vi "Set_PS1_15V_in_Series.vi"(3 "error in":errorcluster) -> (10 "error out":errorcluster)   [LabVIEW 2015]
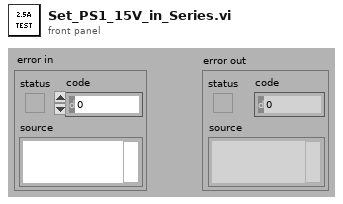
[diagram p1: front panel]
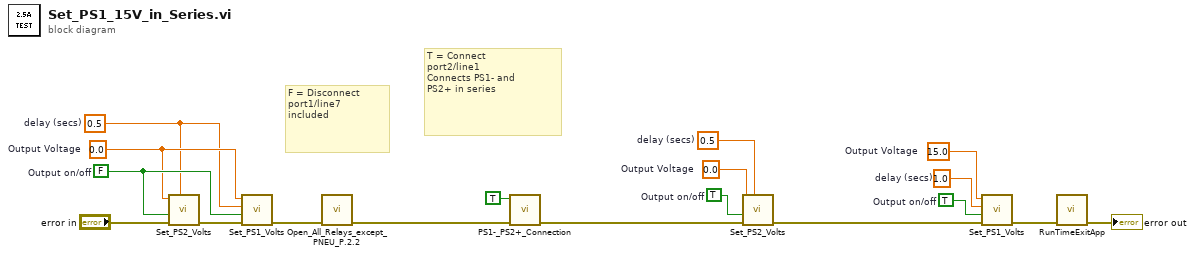
[diagram p0: block diagram]
diagram:
  w3 = TRUE  # Output on/off
  w4 = 0.5  # delay (secs)
  w5 = 0.0  # Output Voltage
  w12 = TRUE  # Output on/off
  w11 = 1.0  # delay (secs)
  w10 = 15.0  # Output Voltage
  w14 = 0.0  # Output Voltage
  w13 = 0.5  # delay (secs)
  w15 = FALSE  # Output on/off
  # "T = Connect\nport2/line1\nConnects PS1- and\nPS2+ in series"
  # "F = Disconnect\nport1/line7\nincluded"
  n1 = call "Set_PS2_Volts.vi"("delay (secs)"=w13, "error in"="error in", "Output on/off"=w15, "Output Voltage"=w14) -> ("error out"=w16:errorcluster)  [unwired: 5 in, 2 out]
  n2 = call "Set_PS1_Volts.vi"("error in"=w16, "Output on/off"=w15, "delay (secs)"=w13, "Output Voltage"=w14) -> ("error out"=w7:errorcluster)  [unwired: 5 in, 2 out]
  n3 = call "Open_All_Relays_except_PNEU_P.2.2.vi"("error in"=w7) -> ("error out"=w6:errorcluster)  [unwired: 9 in]
  n4 = call "PS1-_PS2+_Connection.vi"("On/Off"=TRUE, "error in"=w6) -> ("error out"=w2:errorcluster)  [unwired: 8 in]
  n5 = call "Set_PS2_Volts.vi"("delay (secs)"=w4, "error in"=w2, "Output on/off"=w3, "Output Voltage"=w5) -> ("error out"=w1:errorcluster)  [unwired: 5 in, 2 out]
  n6 = call "Set_PS1_Volts.vi"("error in"=w1, "Output on/off"=w12, "delay (secs)"=w11, "Output Voltage"=w10) -> ("error out"=w9:errorcluster)  [unwired: 5 in, 2 out]
  n7 = call "RunTimeExitApp.vi"("error in (no error)"=w9) -> ("error out"=→"error out":errorcluster)  [unwired: 10 in]
